vi "SW_Shape_Conditions_Array_after_Loading.vi"(2 "error in (no error)":errorcluster, 3 "Conditions presets GZipped in":T1) -> (0 "error out":errorcluster, 1 "Conditions presets array out":T2 {"Specifier(s)"."Validity criteria(s)"."Validity value" min=0.0 step=0.1 format="%.2g"; "Specifier(s)"."Value" step=1.0 format="%#.2g"})   [LabVIEW 2018, in "Common_Resources.lvlib"]
uses:
  SubVi's/Controls/CTL_Conditions_Array.ctl
  SubVi's/Controls/CTL_Conditions_Cluster.ctl
  SubVi's/Controls/CTL_Condition_type.ctl
  SubVi's/Controls/CTL_Comparison_type.ctl
  SubVi's/Controls/CTL_Validity_check_criteria.ctl
  SubVi's/Controls/CTL_Response_info.ctl
  SubVi's/Controls/CTL_Condition_response_type.ctl
  SubVi's/Controls/CTL_Reponse_port_info.ctl
  SubVi's/Controls/CTL_Conditions_GZippped_string.ctl
  Common_Resources.lvlib
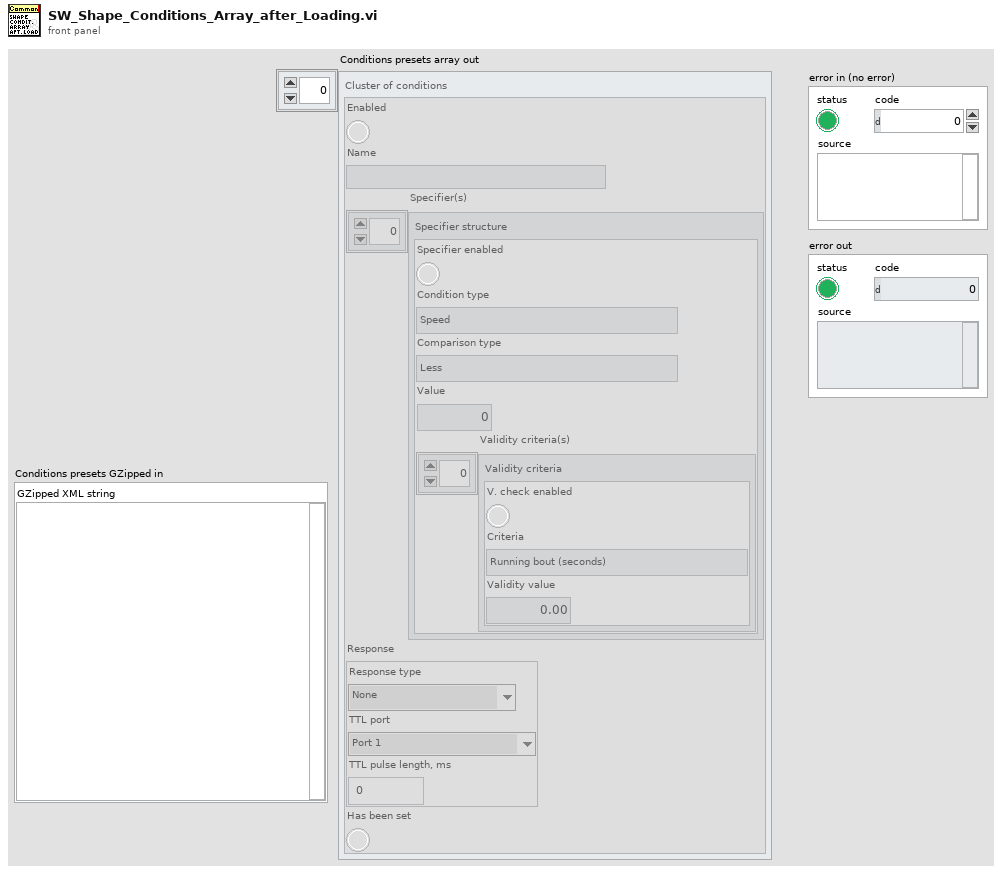
[diagram p1: front panel]
types:
  T1 = typedef "Common_Resources.lvlib/CTL_Conditions_GZippped_string.ctl" = cluster{"GZipped XML string":string}
  T2 = typedef "Common_Resources.lvlib/CTL_Conditions_Array.ctl" = T3[]
  T3 = typedef "Common_Resources.lvlib/CTL_Conditions_Cluster.ctl" = cluster{"Enabled":bool, "Name":string, "Specifier(s)":cluster{"Specifier enabled":bool, "Condition type":T4, "Comparison type":T5, "Value":dbl, "Validity criteria(s)":cluster{"V. check enabled":bool, "Criteria":T6, "Validity value":dbl}[]}[], "Response":T7, "Has been set":bool}
  T4 = typedef "Common_Resources.lvlib/CTL_Condition_type.ctl" = enum16{"Speed", "Zone", "Angle to wall"}
  T5 = typedef "Common_Resources.lvlib/CTL_Comparison_type.ctl" = enum16{"Less", "Less or Equal", "Equal", "Greater or Equal", "Greater", "Not Equal"}
  T6 = typedef "Common_Resources.lvlib/CTL_Validity_check_criteria.ctl" = enum16{"Running bout (seconds)", "Running bout (meters)"}
  T7 = typedef "Common_Resources.lvlib/CTL_Response_info.ctl" = cluster{"Response type":T8, "TTL port":T9, "TTL pulse length, ms":dbl}
  T8 = typedef "Common_Resources.lvlib/CTL_Condition_response_type.ctl" = enum16{"None", "Air puff", "Liquid reward", "TTL pulse", "TTL pulse (ubr)", "TTL signal"}
  T9 = typedef "Common_Resources.lvlib/CTL_Reponse_port_info.ctl" = enum16{"Port 1", "Port 2", "Port 3", "Port 4"}
  T10 = cluster{"Boolean Round":bool, "code":i32, "source":string}
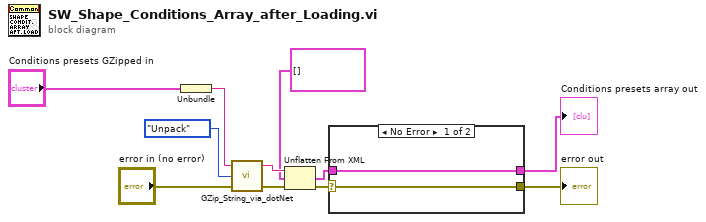
[diagram p0: block diagram]
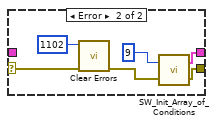
[diagram p2: hidden frame]
diagram:
  n1 = Unbundle("Conditions presets GZipped in") -> ("GZipped XML string"=w8:string)
  n2 = call "GZip_String_via_dotNet.vi"("error in (no error)"="error in (no error)", "Action"=enum16{"Pack", "Unpack"}."Unpack", "String Input"=w8) -> ("error out"=w5:errorcluster, "String Output (GZipped/UnGZipped)"=w7:string)  [unwired: 1 out]
  n3 = Unflatten From XML(xml string=w7, type=T2 [] ("Conditions presets array"), error in (no error)=w5) -> (value=w3:T2, error out=w2:errorcluster)
  n4 = case shown="No Error" w2 {
    selector: w2 -> [w13 w17]
    tunnel: [w13 w15] -> w11
    tunnel: [w12 w18] -> w10
    tunnel: w3 -> [w12 _]
    frame No Error {
    }
    frame Error {
      n5 = call <vilib>:"Clear Errors.vi"("error in (no error)"=w17, "specific error code to clear (0: all)"=1102) -> ("error out"=w16:errorcluster)  [unwired: 4 in, 1 out]
      n6 = call "SW_Init_Array_of_Conditions.vi"("error in (no error)"=w16, "Array size"=9) -> ("error out"=w15:T10, "Array of conditions"=w18:T2)
    }
  }
  "Conditions presets array out" <- w10
  "error out" <- w11
